vi "decodeStream.vi"(8 "error in (no error)":errorcluster, 9 "beginIndex":i32, 10 "binary stream":u8[](array[numeric]), 11 "tBSONJavaScript in":refnum<class "tBSONJavaScript.lvclass">) -> (0 "error out":errorcluster, 1 "endIndex":i32, 2 "binary stream out":u8[](array[numeric]), 3 "tBSONJavaScript out":refnum<class "tBSONJavaScript.lvclass">)   [LabVIEW 2013, in "BSON.lvlib" / "tBSONJavaScript.lvclass"]
uses:
  tBSONJavaScript.lvclass
  tBSONElement/tBSONElement.lvclass
  setScript.vi
  BSON.lvlib
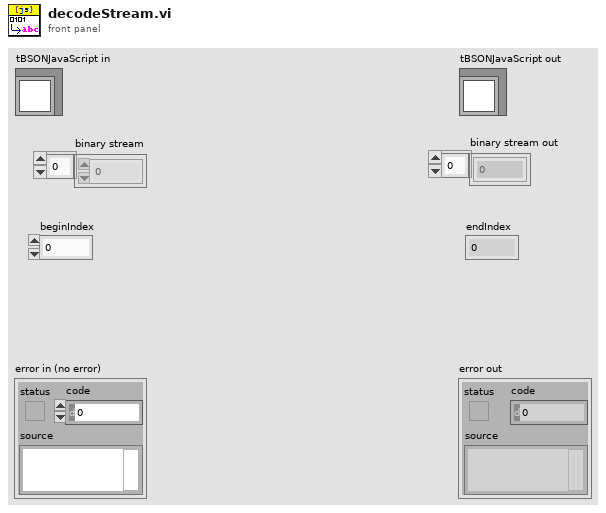
[diagram p1: front panel]
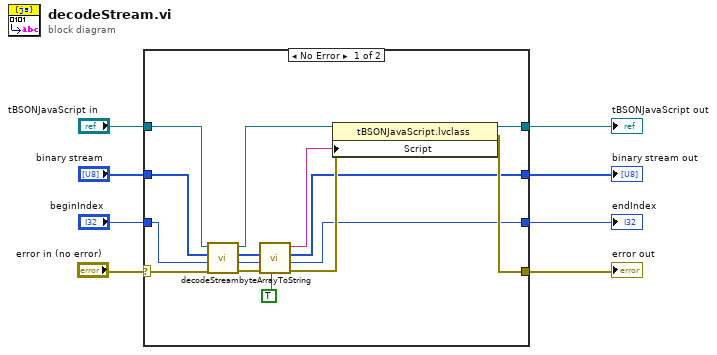
[diagram p0: block diagram]
diagram:
  n1 = case shown="No Error" "error in (no error)" {
    selector: "error in (no error)" -> [w23 w27]
    tunnel: [w18 w27] -> w1
    tunnel: "beginIndex" -> [w21 w26]
    tunnel: [w11 w26] -> w3
    tunnel: "binary stream" -> [w20 w25]
    tunnel: [w12 w25] -> w2
    tunnel: "tBSONJavaScript in" -> [w22 w24]
    tunnel: [w17 w24] -> w7
    frame No Error {
      n2 = call-parent "decodeStream.vi"("error in (no error)"=w23, "beginIndex"=w21, "binary stream"=w20, "tBSONElement in"=w22) -> ("error out"=w16:errorcluster, "endIndex"=w14:i32, "binary stream out"=w13:u8[], "tBSONElement out"=w19:refnum<class "tBSONJavaScript.lvclass">)  [unwired: 4 in]
      n3 = call "byteArrayToString.vi"("lengthPrepended"=TRUE, "error in (no error)"=w16, "startIndex"=w14, "ByteArrayIn"=w13) -> ("error out"=w15:errorcluster, "endIndex"=w11:i32, "ByteArrayOut"=w12:u8[], "String"=w10:string)  [unwired: 4 in]
      n4 = property class="tBSONJavaScript.lvclass"(reference=w19, error in=w15, "Script"=w10) -> (reference out=w17:refnum<class "tBSONJavaScript.lvclass">, error out=w18:errorcluster)
    }
    frame Error {
    }
  }
  "error out" <- w1
  "tBSONJavaScript out" <- w7
  "binary stream out" <- w2
  "endIndex" <- w3
